vi "Deinit.vi"(8 "error in":errorcluster, 11 "VISA Interface in":refnum<class "VISA Interface.lvclass">) -> (0 "error out":errorcluster, 3 "VISA Interface out":refnum<class "VISA Interface.lvclass">)   [LabVIEW 2020, in "Plugin Instrument Driver.lvlib" / "VISA Interface.lvclass"]
doc: "Close VISA reference"
uses:
  VISA Interface.lvclass
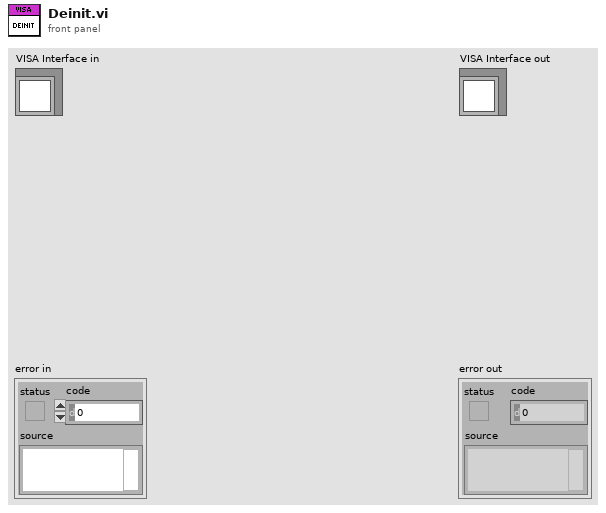
[diagram p1: front panel]
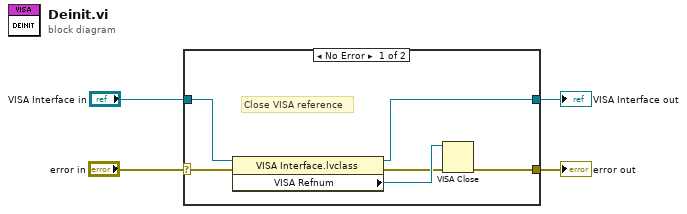
[diagram p0: block diagram]
diagram:
  n1 = case shown="No Error" "error in" {
    selector: "error in" -> [w10 w11]
    tunnel: "VISA Interface in" -> [w9 w12]
    tunnel: [w6 w11] -> w2
    tunnel: [w5 w12] -> w1
    frame No Error {
      # "Close VISA reference"
      n2 = property class="VISA Interface.lvclass"(reference=w9, error in=w10) -> (reference out=w5:refnum<class "VISA Interface.lvclass">, error out=w7:errorcluster, "VISA Refnum"=w8:refnum<visa-resource-name>)
      n3 = VISA Close(VISA resource name=w8, error in (no error)=w7) -> (error out=w6:errorcluster)
    }
    frame Error {
    }
  }
  "error out" <- w2
  "VISA Interface out" <- w1
